vi "Set Channel Filter.vi"(6 "Filter enable?":bool, 8 "error in (no error)":errorcluster, 9 "Cutoff frequency in Hz":dbl, 10 "Channel":u16(ring) items=["A1"=0, "A2"=1, "A3"=2, "A4"=3, "A5"=4, "A6"=5, "A7"=6, "A8"=7, "A9"=8, "A10"=9, "K1"=200, "K2"=201, "K3"=202, "K4"=203, "FA1"=204, "FA2"=205, "FA3"=206, "FA4"=207], 11 "VISA resource name":refnum<visa-resource-name>) -> (0 "error out":errorcluster, 3 "VISA resource name out":refnum<visa-resource-name>)   [LabVIEW 2017, in "Sefram DAS220.lvlib"]
doc: "Set a low-pass filter on a channel. Cutoff frequency at 0 Hz means filter disabled."
uses:
  <instrlib>/Sefram DAS220/Sefram DAS220.lvlib
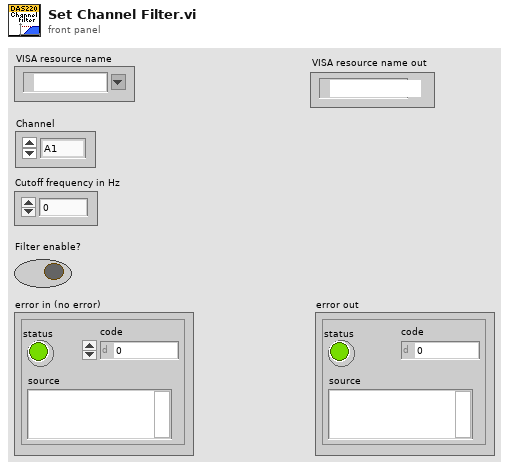
[diagram p1: front panel]
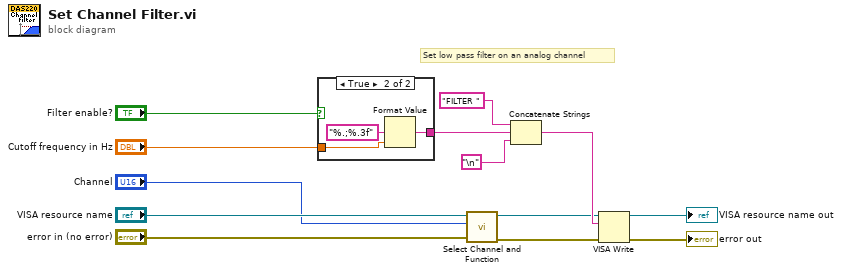
[diagram p0: block diagram]
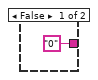
[diagram p2: hidden frame]
diagram:
  # "Set low pass filter on an analog channel"
  n1 = case shown="True" "Filter enable?" {
    tunnel: "Cutoff frequency in Hz" -> [_ w16]
    tunnel: ["0" ("output string") w15] -> w7
    frame False {
    }
    frame True {
      n2 = Format Value(format string="%.;%.3f", value (0)=w16) -> (output string=w15:string)  [unwired: 1 in]
    }
  }
  n3 = call <instrlib>:"Select Channel and Function.vi"("error in (no error)"="error in (no error)", "Channel"="Channel", "VISA resource name"="VISA resource name") -> ("error out"=w3:errorcluster, "VISA resource name out"=w4:refnum<visa-resource-name>)  [unwired: 7 in]
  n4 = Concatenate Strings("FILTER " ("string"), w7, "\n") -> (w13:string)
  n5 = VISA Write(VISA resource name=w4, write buffer=w13, error in (no error)=w3) -> (VISA resource name out=→"VISA resource name out":refnum<visa-resource-name>, error out=→"error out":errorcluster)  [unwired: 1 out]
